vi "Display.vi"(8 "error in":errorcluster, 10 "Sub Panel":refnum<vi>, 11 "IDatabase UI in":refnum<class "IDatabase UI.lvclass">) -> (0 "error out":errorcluster, 3 "IDatabase UI out":refnum<class "IDatabase UI.lvclass">)   [LabVIEW 2023, in "IDatabase UI.lvlib" / "IDatabase UI.lvclass"]
uses:
  IDatabase UI.lvclass
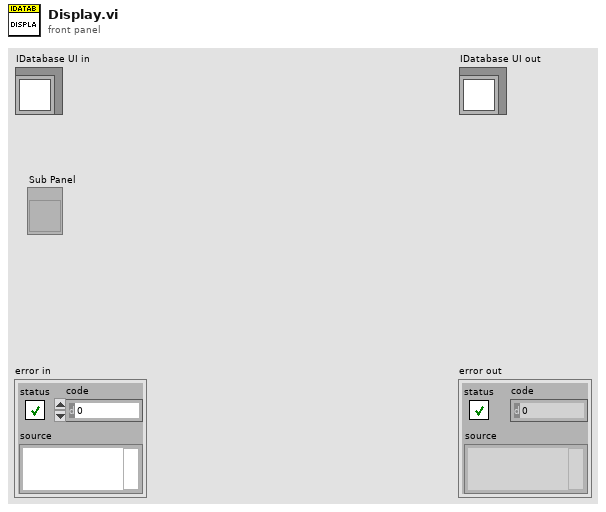
[diagram p1: front panel]
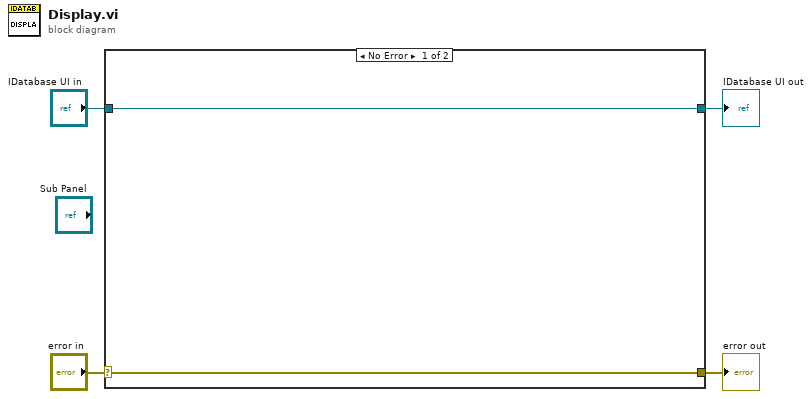
[diagram p0: block diagram]
diagram:
  n1 = case shown="No Error" "error in" {
    selector: "error in" -> [w5 w8]
    tunnel: [w5 w8] -> w3
    tunnel: [w6 w7] -> w1
    tunnel: "IDatabase UI in" -> [w6 w7]
    frame No Error {
    }
    frame Error {
    }
  }
  "error out" <- w3
  "IDatabase UI out" <- w1
